vi "SeCrTs-DO State Ref Disable.vi"(10 "DO ref in":refnum<vi>[](array[refnum]), 11 "Disabled":T1(ring)) -> ()   [LabVIEW 2022 SP3]
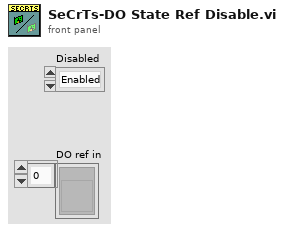
[diagram p1: front panel]
types:
  T1 = enum8{"Enabled", "Disabled", "Disabled and Grayed Out"}
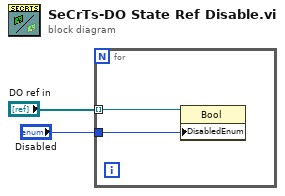
[diagram p0: block diagram]
diagram:
  n1 = for {
    tunnel: "DO ref in" -> [w4] mode=indexing
    tunnel: "Disabled" -> [w3]
    n2 = property class="Bool"(reference=w4, "DisabledEnum"=w3) -> ()  [unwired: 1 in, 2 out]
  }
